vi "Limit Alarm Server.vi"() -> ()   [LabVIEW 2019, in "OPC UA Demo.lvlib"]
doc: "Demonstrates the use of the <B>OPC UA Alarms and Conditions</B> functionality as an OPC UA server."
uses:
  OPC UA Demo.lvlib
  <vilib>/OPCUA/controls/Data Type.ctl
  <vilib>/OPCUA/controls/NodeId.ctl
  <vilib>/OPCUA/controls/Historical Access.ctl
  <vilib>/OPCUA/server/Add Exclusive Level Alarm.vi
  <vilib>/OPCUA/server/Add Nonexclusive Deviation Alarm.vi
  <vilib>/OPCUA/server/Write Double.vi
  <vilib>/OPCUA/NI OPC UA Server.lvlib
  <vilib>/ptbypt/NI_PtbyPt.lvlib
panel:
  in  "source node amplitude":dbl=80.0
  in  "queue size (1000)":u32=1000
  in  "low limit":dbl=40.0
  in  "low low limit":dbl=20.0
  in  "high limit":dbl=60.0
  in  "high high limit":dbl=80.0
  in  "set point value":dbl=50.0
  in  "low low limit":dbl=-30.0 format="%#_13g"
  in  "low limit":dbl=-10.0 format="%#_13g"
  in  "high limit":dbl=10.0 format="%#_13g"
  in  "high high limit":dbl=30.0 format="%#_13g"
  in  "stop":bool
  out "source node value":dbl(graph)
  out "server endpoint URL":string
  # "Overview: Demonstrates the use of the OPC UA Alarms and Conditions functionality as an OPC UA server.\nRequirements: \n1. LabVIEW OPC UA Toolkit\n2. Run this VI on RT targets or Windows\nInstructions:\n1. Adjust queue size to change the buffer size of history event data.\n2. Run the VI.\n3. Run Limit Alarm Client.vi in OPC UA Demo.lvproj."
  # "Level Alarm"
  # "Deviation Alarm"
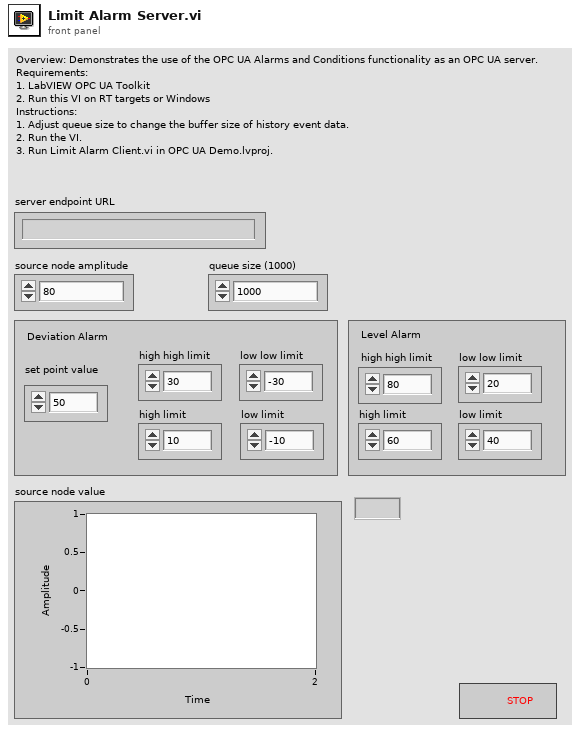
[diagram p1: front panel]
types:
  T1 = typedef "Historical Access.ctl" = cluster{"enable":bool, "queue size (1000)":u32}
  T2 = typedef "NodeId.ctl" = string
  T3 = cluster{"condition name":string, "source node ID":T2, "setpoint node ID":T2, "limit":cluster{"high high limit":dbl, "high limit":dbl, "low limit":dbl, "low low limit":dbl}, "description":string}
  T4 = typedef "Data Type.ctl" = u16
  T5 = cluster{"name":string, "data type":T4, "access level":u16, "description":string}
  T6 = cluster{"condition name":string, "source node ID":T2, "limit":cluster{"high high limit":dbl, "high limit":dbl, "low limit":dbl, "low low limit":dbl}, "description":string}
  T7 = typedef "OPC UA Server Refnum.ctl" = refnum<k21>
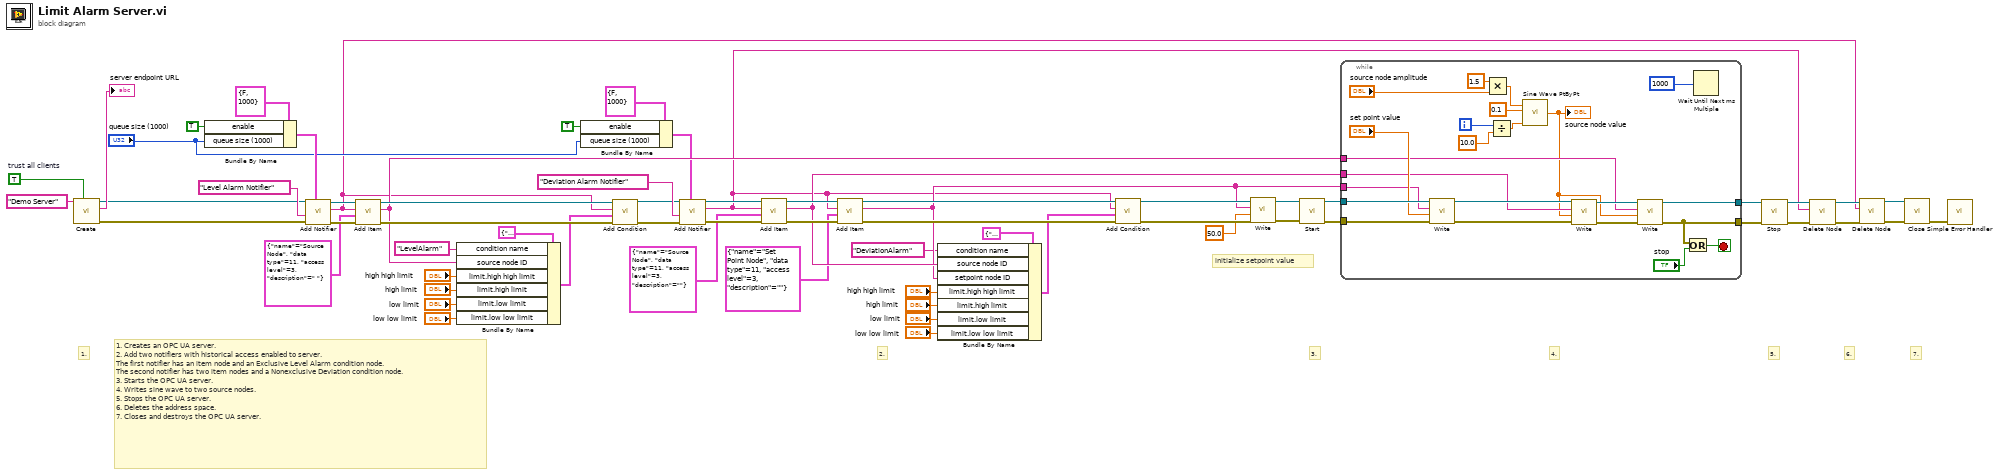
[diagram p0: block diagram]
diagram:
  w1 = TRUE  # trust all clients
  # "initialize setpoint value"
  # "7."
  # "6."
  # "5."
  # "4."
  # "3."
  # "2."
  # "1."
  # "1. Creates an OPC UA server.\n2. Add two notifiers with historical access enabled to server.\nThe first notifier has an item node and an Exclusive Level Alarm condition node.\nThe second notifier has two item nodes and a Nonexclusive Deviation condition node.\n3. Starts the OPC UA server.\n4. Writes sine wave to two source nodes.\n5. Stops the OPC UA server.\n6. Deletes the address space.\n7. Closes and destroys the OPC UA server."
  n1 = call <vilib>:"Create.vi"("trust all clients (F)"=w1, "OPC UA server name"="Demo Server") -> ("error out"=w31:errorcluster, "server endpoint URL"=→"server endpoint URL":string, "OPC UA server refnum out"=w30:T7)  [unwired: 7 in]
  n2 = Bundle By Name(cluster=T1 {"enable"=FALSE, "queue size (1000)"=1000} ("historical access"), "enable"=TRUE, "queue size (1000)"="queue size (1000)") -> (w21:T1)
  n3 = call <vilib>:"Add Notifier.vi"("historical access"=w21, "error in (no error)"=w31, "notifier name"="Level Alarm Notifier" ("folder name"), "OPC UA server refnum in"=w30) -> ("error out"=w37:errorcluster, "notifier node ID"=w8:T2, "OPC UA server refnum out"=w38:T7)  [unwired: 3 in, 1 out]
  n4 = call <vilib>:"Add Item.vi"("error in (no error)"=w37, "item"=T5 {"name"="Source Node", "data type"=11, "access level"=3, "description"=" "}, "parent folder node ID"=w8, "OPC UA server refnum in"=w38) -> ("error out"=w40:errorcluster, "item node ID"=w28:T2, "OPC UA server refnum out"=w41:T7)  [unwired: 3 in, 1 out]
  n5 = Bundle By Name(cluster=T6 {"condition name"="", "source node ID"="", "limit"={"high high limit"=80.0, "high limit"=60.0, "low limit"=40.0, "low low limit"=20.0}, "description"=""} ("property"), "condition name"="LevelAlarm", "source node ID"=w28, "limit.high high limit"="high high limit", "limit.high limit"="high limit", "limit.low limit"="low limit", "limit.low low limit"="low low limit") -> (w39:T6)
  n6 = Bundle By Name(cluster=T1 {"enable"=FALSE, "queue size (1000)"=1000} ("historical access"), "enable"=TRUE, "queue size (1000)"="queue size (1000)") -> (w19:T1)
  n7 = call-poly <vilib>:"Add Condition.vi"("error in (no error)"=w40, "property"=w39, "notifier node ID"=w8, "OPC UA server refnum in"=w41) -> ("error out"=w29:errorcluster, "OPC UA server refnum out"=w3:T7)  [unwired: 4 in, 2 out]
  n8 = call <vilib>:"Add Notifier.vi"("historical access"=w19, "error in (no error)"=w29, "notifier name"="Deviation Alarm Notifier" ("folder name"), "OPC UA server refnum in"=w3) -> ("error out"=w51:errorcluster, "notifier node ID"=w7:T2, "OPC UA server refnum out"=w52:T7)  [unwired: 3 in, 1 out]
  n9 = call <vilib>:"Add Item.vi"("error in (no error)"=w51, "item"=T5 {"name"="Source Node", "data type"=11, "access level"=3, "description"=""}, "parent folder node ID"=w7, "OPC UA server refnum in"=w52) -> ("error out"=w60:errorcluster, "item node ID"=w49:T2, "OPC UA server refnum out"=w50:T7)  [unwired: 3 in, 1 out]
  n10 = call <vilib>:"Add Item.vi"("error in (no error)"=w60, "item"=T5 {"name"="Set Point Node", "data type"=11, "access level"=3, "description"=""}, "parent folder node ID"=w7, "OPC UA server refnum in"=w50) -> ("error out"=w59:errorcluster, "item node ID"=w23:T2, "OPC UA server refnum out"=w61:T7)  [unwired: 3 in, 1 out]
  n11 = Bundle By Name(cluster=T3 {"condition name"="", "source node ID"="", "setpoint node ID"="", "limit"={"high high limit"=80.0, "high limit"=60.0, "low limit"=40.0, "low low limit"=20.0}, "description"=""} ("property"), "condition name"="DeviationAlarm", "source node ID"=w49, "setpoint node ID"=w23, "limit.high high limit"="high high limit", "limit.high limit"="high limit", "limit.low limit"="low limit", "limit.low low limit"="low low limit") -> (w48:T3)
  n12 = call-poly <vilib>:"Add Condition.vi"("error in (no error)"=w59, "property"=w48, "notifier node ID"=w7, "OPC UA server refnum in"=w61) -> ("error out"=w25:errorcluster, "OPC UA server refnum out"=w27:T7)  [unwired: 4 in, 2 out]
  n13 = call-poly <vilib>:"Write.vi"("error in (no error)"=w25, "value"=50.0, "node ID"=w23, "OPC UA server refnum in"=w27) -> ("error out"=w24:errorcluster, "OPC UA server refnum out"=w26:T7)  [unwired: 5 in, 1 out]
  n14 = call <vilib>:"Start.vi"("error in (no error)"=w24, "OPC UA server refnum in"=w26) -> ("error out"=w43:errorcluster, "OPC UA server refnum out"=w58:T7)  [unwired: 7 in, 1 out]
  n15 = while {
    tunnel: w58 -> [w83]
    tunnel: w43 -> [w86]
    tunnel: w49 -> [w76]
    tunnel: [w78] -> w47
    tunnel: [w66] -> w46
    tunnel: w23 -> [w81]
    tunnel: w28 -> [w77]
    i -> [w73]
    stop <- w67 stop-if-true
    n16 = call-poly <vilib>:"Write.vi"("error in (no error)"=w86, "value"="set point value", "node ID"=w81, "OPC UA server refnum in"=w83) -> ("error out"=w85:errorcluster, "OPC UA server refnum out"=w84:T7)  [unwired: 5 in, 1 out]
    n17 = Multiply(x=1.5 ("y"), y="source node amplitude") -> (x*y=w69:dbl)
    n18 = Divide(x=w73, y=10.0 ("frequency")) -> (x/y=w75:dbl)
    n19 = call <vilib>:"Sine Wave PtByPt.vi"("time"=w75, "frequency"=0.1, "amplitude"=w69) -> ("sine wave"=w72:dbl)  [unwired: 1 in]
    "source node value" <- w72
    n20 = call-poly <vilib>:"Write.vi"("error in (no error)"=w85, "value"=w72, "node ID"=w76, "OPC UA server refnum in"=w84) -> ("error out"=w79:errorcluster, "OPC UA server refnum out"=w80:T7)  [unwired: 5 in, 1 out]
    n21 = call-poly <vilib>:"Write.vi"("error in (no error)"=w79, "value"=w72, "node ID"=w77, "OPC UA server refnum in"=w80) -> ("error out"=w66:errorcluster, "OPC UA server refnum out"=w78:T7)  [unwired: 5 in, 1 out]
    n22 = Or(x=w66, y="stop") -> (x .or. y?=w67:bool)
    n23 = Wait Until Next ms Multiple(millisecond multiple=u32 1000) -> ()  [unwired: 1 out]
  }
  n24 = call <vilib>:"Stop.vi"("error in (no error)"=w46, "OPC UA server refnum in"=w47) -> ("error out"=w45:errorcluster, "OPC UA server refnum out"=w44:T7)  [unwired: 8 in]
  n25 = call <vilib>:"Delete Node.vi"("error in (no error)"=w45, "node ID"=w7, "OPC UA server refnum in"=w44) -> ("error out"=w12:errorcluster, "OPC UA server refnum out"=w11:T7)  [unwired: 7 in]
  n26 = call <vilib>:"Delete Node.vi"("error in (no error)"=w12, "node ID"=w8, "OPC UA server refnum in"=w11) -> ("error out"=w10:errorcluster, "OPC UA server refnum out"=w9:T7)  [unwired: 7 in]
  n27 = call <vilib>:"Close.vi"("error in (no error)"=w10, "OPC UA server refnum in"=w9) -> ("error out"=w57:errorcluster)  [unwired: 9 in]
  n28 = call <vilib>:"Simple Error Handler.vi"("error in (no error)"=w57) -> ()  [unwired: 4 in, 5 out]
